vi "PC_Host_App_Boucle_Non_Deterministe.vi"() -> ()   [LabVIEW 2019]
panel:
  in  "stop":bool
  out "Waveform Chart":dbl(graph)
  in  "Boolean":bool
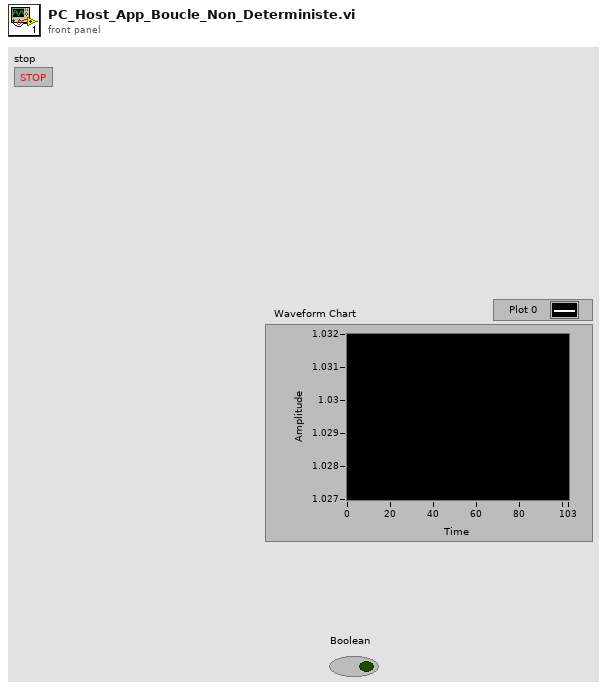
[diagram p1: front panel]
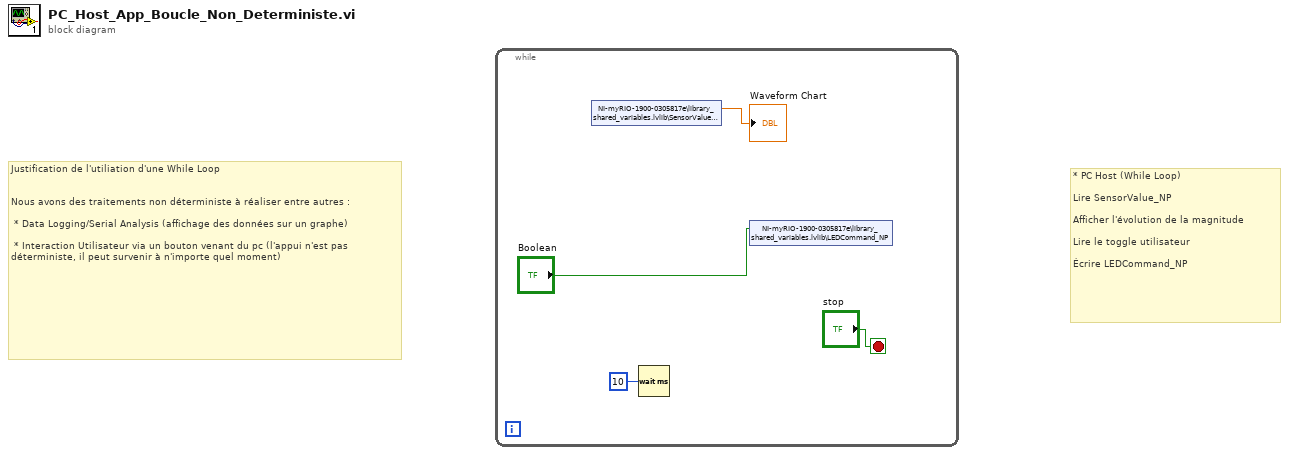
[diagram p0: block diagram]
diagram:
  # "* PC Host (While Loop)\n\nLire SensorValue_NP\n\nAfficher l'évolution de la magnitude\n\nLire le toggle utilisateur\n\nÉcrire LEDCommand_NP"
  # "Justification de l'utiliation d'une While Loop   \n\n\nNous avons des traitements non déterministe à réaliser entre autres :\n\n * Data Logging/Serial Analysis (affichage des données sur un graphe)\n\n * Interaction Utilisateur via un bouton venant du pc (l'appui n'est pas déterministe, il peut survenir à n'importe quel moment)"
  n1 = while {
    stop <- "stop" stop-if-true
    n2 = shared-variable "NI-myRIO-1900-0305817e\\library_shared_variables.lvlib\\SensorValue_NP"() -> (→"Waveform Chart":dbl)  [unwired: 1 in, 1 out]
    n3 = Wait (ms)(milliseconds to wait=u32 10) -> ()  [unwired: 1 out]
    n4 = shared-variable "NI-myRIO-1900-0305817e\\library_shared_variables.lvlib\\LEDCommand_NP"("Boolean") -> ()  [unwired: 1 in, 1 out]
  }
